vi "cast_meta_idx_toFXP.vi"(8 "error in":errorcluster, 10 "cs-traj-data-in":dbl[](array[numeric])) -> (0 "error out":errorcluster, 2 "cs-traj-data-out":fxp<+/-,16,5>[](array[numeric]))   [LabVIEW 2019]
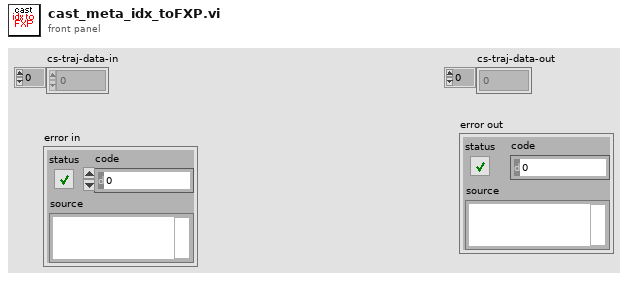
[diagram p1: front panel]
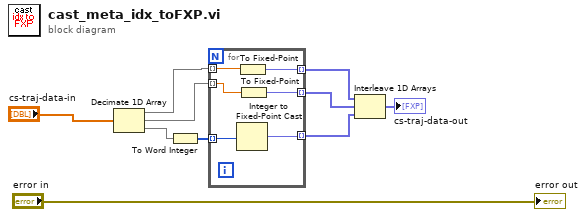
[diagram p0: block diagram]
diagram:
  n1 = Decimate 1D Array("cs-traj-data-in") -> (w5:dbl[], w6:dbl[], w4:dbl[])
  n2 = To Word Integer(number=w4) -> (16bit integer=w7:i16[])
  n3 = for {
    tunnel: w5 -> [w16] mode=indexing
    tunnel: w6 -> [w15] mode=indexing
    tunnel: [w14] -> w9 mode=indexing
    tunnel: [w13] -> w8 mode=indexing
    tunnel: w7 -> [w12] mode=indexing
    tunnel: [w11] -> w10 mode=indexing
    n4 = Integer to Fixed-Point Cast(integer=w12) -> (fixed-point=w11:fxp<+/-,16,5>)  [unwired: 1 in]
    n5 = To Fixed-Point(number=w16) -> (fixed-point=w13:fxp<+/-,16,5>)  [unwired: 1 in]
    n6 = To Fixed-Point(number=w15) -> (fixed-point=w14:fxp<+/-,16,5>)  [unwired: 1 in]
  }
  n7 = Interleave 1D Arrays(w8, w9, w10) -> (→"cs-traj-data-out":fxp<+/-,16,5>[])
  "error out" <- "error in"
